vi "DealData.vi"(2 "mbfDealData":bool, 3 "ArrayIn":u8[](array[numeric]) format="0x%x") -> (0 "mu08BufSize":u8, 1 "Result":string[](array[string]))   [LabVIEW 2011]
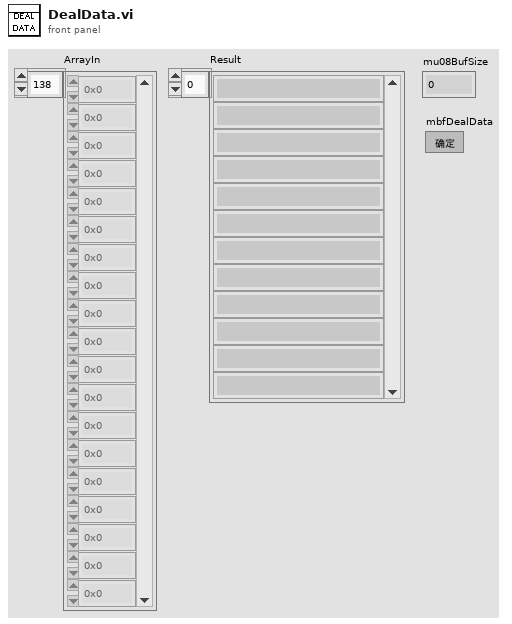
[diagram p1: front panel]
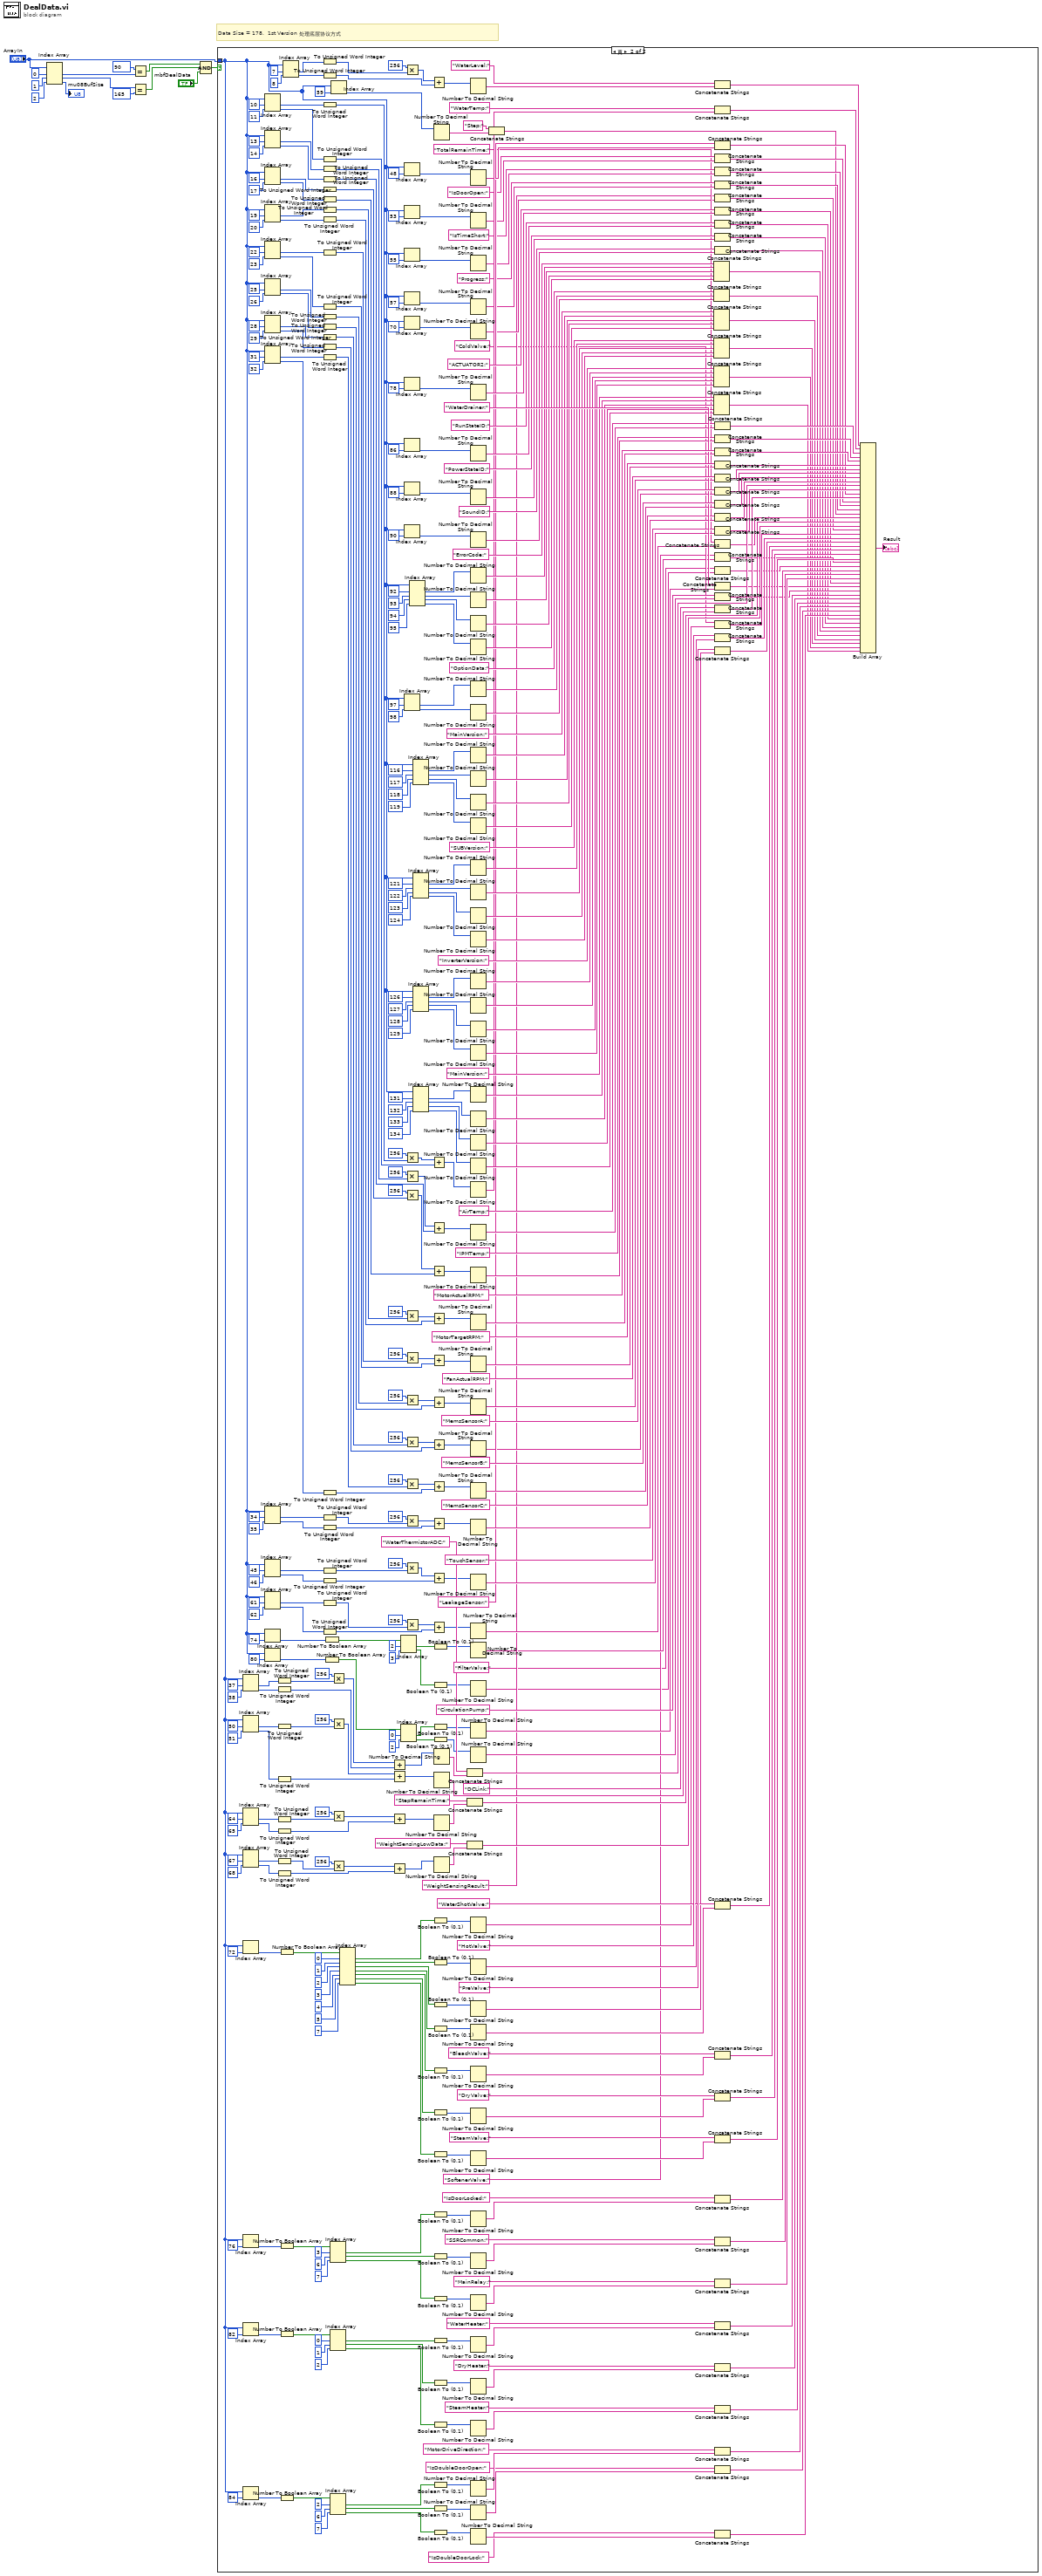
[diagram p0: block diagram]
diagram:
  # "Data Size = 178,  1st Version 处理底层协议方式"
  n1 = Index Array(array="ArrayIn", index #1=0 ("索引"), index #2=1 ("索引"), index #3=2 ("索引")) -> (element #1=w11:u8, element #2=w8:u8, element #3=→"mu08BufSize":u8)
  n2 = Equal?(x=u8 90, y=w11) -> (x = y?=w7:bool)
  n3 = Equal?(x=w8, y=u8 165) -> (x = y?=w6:bool)
  n4 = Compound Arithmetic op=AND(w7, w6, "mbfDealData") -> (w4:bool)
  n5 = case shown="真" w4 {
    tunnel: "ArrayIn" -> [_ w65]
    frame False {
    }
    frame True {
      n6 = Index Array(array=w65, index #1=37 ("索引"), index #2=38 ("索引")) -> (element #1=w361:u8, element #2=w360:u8)
      n7 = Index Array(array=w65, index #1=50 ("索引"), index #2=51 ("索引")) -> (element #1=w339:u8, element #2=w338:u8)
      n8 = Index Array(array=w65, index #1=64 ("索引"), index #2=65 ("索引")) -> (element #1=w305:u8, element #2=w304:u8)
      n9 = Index Array(array=w65, index #1=67 ("索引"), index #2=68 ("索引")) -> (element #1=w294:u8, element #2=w293:u8)
      n10 = Index Array(array=w65, index=72 ("索引")) -> (element=w287:u8)
      n11 = Index Array(array=w65, index=76 ("索引")) -> (element=w259:u8)
      n12 = Index Array(array=w65, index=82 ("索引")) -> (element=w224:u8)
      n13 = Index Array(array=w65, index=84 ("索引")) -> (element=w173:u8)
      n14 = Index Array(array=w65, index #1=10 ("索引"), index #2=11 ("索引")) -> (element #1=w460:u8, element #2=w457:u8)
      n15 = Index Array(array=w65, index #1=13 ("索引"), index #2=14 ("索引")) -> (element #1=w445:u8, element #2=w444:u8)
      n16 = Index Array(array=w65, index #1=16 ("索引"), index #2=17 ("索引")) -> (element #1=w426:u8, element #2=w425:u8)
      n17 = Index Array(array=w65, index #1=19 ("索引"), index #2=20 ("索引")) -> (element #1=w427:u8, element #2=w424:u8)
      n18 = Index Array(array=w65, index #1=22 ("索引"), index #2=23 ("索引")) -> (element #1=w414:u8, element #2=w413:u8)
      n19 = Index Array(array=w65, index #1=25 ("索引"), index #2=26 ("索引")) -> (element #1=w403:u8, element #2=w402:u8)
      n20 = Index Array(array=w65, index #1=28 ("索引"), index #2=29 ("索引")) -> (element #1=w392:u8, element #2=w391:u8)
      n21 = Index Array(array=w65, index #1=31 ("索引"), index #2=32 ("索引")) -> (element #1=w372:u8, element #2=w373:u8)
      n22 = Index Array(array=w65, index #1=34 ("索引"), index #2=35 ("索引")) -> (element #1=w369:u8, element #2=w370:u8)
      n23 = Index Array(array=w65, index #1=45 ("索引"), index #2=46 ("索引")) -> (element #1=w349:u8, element #2=w348:u8)
      n24 = Index Array(array=w65, index #1=61 ("索引"), index #2=62 ("索引")) -> (element #1=w316:u8, element #2=w315:u8)
      n25 = Index Array(array=w65, index=74 ("索引")) -> (element=w201:u8)
      n26 = Index Array(array=w65, index=80 ("索引")) -> (element=w237:u8)
      n27 = To Unsigned Word Integer(number=w361) -> (unsigned 16bit integer=w365:u16)
      n28 = To Unsigned Word Integer(number=w360) -> (unsigned 16bit integer=w363:u16)
      n29 = To Unsigned Word Integer(number=w339) -> (unsigned 16bit integer=w342:u16)
      n30 = To Unsigned Word Integer(number=w338) -> (unsigned 16bit integer=w341:u16)
      n31 = To Unsigned Word Integer(number=w305) -> (unsigned 16bit integer=w311:u16)
      n32 = To Unsigned Word Integer(number=w304) -> (unsigned 16bit integer=w310:u16)
      n33 = To Unsigned Word Integer(number=w294) -> (unsigned 16bit integer=w300:u16)
      n34 = To Unsigned Word Integer(number=w293) -> (unsigned 16bit integer=w299:u16)
      n35 = Number To Boolean Array(number=w287) -> (Boolean array=w286:bool[])
      n36 = Number To Boolean Array(number=w259) -> (Boolean array=w256:bool[])
      n37 = Number To Boolean Array(number=w224) -> (Boolean array=w223:bool[])
      n38 = Number To Boolean Array(number=w173) -> (Boolean array=w177:bool[])
      n39 = Index Array(array=w65, index #1=7 ("索引"), index #2=8 ("索引")) -> (element #1=w463:u8, element #2=w461:u8)
      n40 = To Unsigned Word Integer(number=w463) -> (unsigned 16bit integer=w464:u16)
      n41 = To Unsigned Word Integer(number=w461) -> (unsigned 16bit integer=w462:u16)
      n42 = To Unsigned Word Integer(number=w460) -> (unsigned 16bit integer=w459:u16)
      n43 = To Unsigned Word Integer(number=w457) -> (unsigned 16bit integer=w456:u16)
      n44 = To Unsigned Word Integer(number=w445) -> (unsigned 16bit integer=w450:u16)
      n45 = To Unsigned Word Integer(number=w444) -> (unsigned 16bit integer=w448:u16)
      n46 = To Unsigned Word Integer(number=w426) -> (unsigned 16bit integer=w440:u16)
      n47 = To Unsigned Word Integer(number=w425) -> (unsigned 16bit integer=w438:u16)
      n48 = To Unsigned Word Integer(number=w427) -> (unsigned 16bit integer=w432:u16)
      n49 = To Unsigned Word Integer(number=w424) -> (unsigned 16bit integer=w430:u16)
      n50 = To Unsigned Word Integer(number=w414) -> (unsigned 16bit integer=w419:u16)
      n51 = To Unsigned Word Integer(number=w413) -> (unsigned 16bit integer=w417:u16)
      n52 = To Unsigned Word Integer(number=w403) -> (unsigned 16bit integer=w408:u16)
      n53 = To Unsigned Word Integer(number=w402) -> (unsigned 16bit integer=w406:u16)
      n54 = To Unsigned Word Integer(number=w392) -> (unsigned 16bit integer=w397:u16)
      n55 = To Unsigned Word Integer(number=w391) -> (unsigned 16bit integer=w395:u16)
      n56 = To Unsigned Word Integer(number=w372) -> (unsigned 16bit integer=w386:u16)
      n57 = To Unsigned Word Integer(number=w373) -> (unsigned 16bit integer=w384:u16)
      n58 = To Unsigned Word Integer(number=w369) -> (unsigned 16bit integer=w377:u16)
      n59 = To Unsigned Word Integer(number=w370) -> (unsigned 16bit integer=w375:u16)
      n60 = To Unsigned Word Integer(number=w349) -> (unsigned 16bit integer=w354:u16)
      n61 = To Unsigned Word Integer(number=w348) -> (unsigned 16bit integer=w352:u16)
      n62 = To Unsigned Word Integer(number=w316) -> (unsigned 16bit integer=w322:u16)
      n63 = To Unsigned Word Integer(number=w315) -> (unsigned 16bit integer=w321:u16)
      n64 = Number To Boolean Array(number=w201) -> (Boolean array=w200:bool[])
      n65 = Number To Boolean Array(number=w237) -> (Boolean array=w236:bool[])
      n66 = Index Array(array=w256, index #1=3 ("索引"), index #2=6 ("索引"), index #3=7 ("索引")) -> (element #1=w254:bool, element #2=w253:bool, element #3=w252:bool)
      n67 = Index Array(array=w223, index #1=0 ("索引"), index #2=1 ("索引"), index #3=2 ("索引")) -> (element #1=w218:bool, element #2=w217:bool, element #3=w184:bool)
      n68 = Index Array(array=w177, index #1=2 ("索引"), index #2=6 ("索引"), index #3=7 ("索引")) -> (element #1=w169:bool, element #2=w168:bool, element #3=w167:bool)
      n69 = Index Array(array=w65, index=59 ("索引")) -> (element=w63:u8)
      n70 = Multiply(x=u16 256, y=w365) -> (x*y=w364:u16)
      n71 = Multiply(x=u16 256, y=w342) -> (x*y=w337:u16)
      n72 = Multiply(x=u16 256, y=w311) -> (x*y=w308:u16)
      n73 = Multiply(x=u16 256, y=w300) -> (x*y=w297:u16)
      n74 = Index Array(array=w286, index #1=0 ("索引"), index #2=1 ("索引"), index #3=2 ("索引"), index #4=3 ("索引"), index #5=4 ("索引"), index #6=5 ("索引"), index #7=7 ("索引")) -> (element #1=w276:bool, element #2=w275:bool, element #3=w274:bool, element #4=w273:bool, element #5=w272:bool, element #6=w209:bool, element #7=w208:bool)
      n75 = Add(x=w364, y=w363) -> (x+y=w362:u16)
      n76 = Add(x=w337, y=w341) -> (x+y=w336:u16)
      n77 = Add(x=w308, y=w310) -> (x+y=w307:u16)
      n78 = Add(x=w297, y=w299) -> (x+y=w296:u16)
      n79 = Index Array(array=w200, index #1=2 ("索引"), index #2=3 ("索引")) -> (element #1=w197:bool, element #2=w196:bool)
      n80 = Index Array(array=w236, index #1=0 ("索引"), index #2=2 ("索引")) -> (element #1=w233:bool, element #2=w232:bool)
      n81 = Index Array(array=w65, index=48 ("索引")) -> (element=w62:u8)
      n82 = Index Array(array=w65, index=53 ("索引")) -> (element=w334:u8)
      n83 = Index Array(array=w65, index=55 ("索引")) -> (element=w331:u8)
      n84 = Index Array(array=w65, index=57 ("索引")) -> (element=w328:u8)
      n85 = Index Array(array=w65, index=70 ("索引")) -> (element=w290:u8)
      n86 = Index Array(array=w65, index=78 ("索引")) -> (element=w239:u8)
      n87 = Index Array(array=w65, index=86 ("索引")) -> (element=w156:u8)
      n88 = Index Array(array=w65, index=88 ("索引")) -> (element=w151:u8)
      n89 = Index Array(array=w65, index=90 ("索引")) -> (element=w144:u8)
      n90 = Index Array(array=w65, index #1=97 ("索引"), index #2=98 ("索引")) -> (element #1=w123:u8, element #2=w122:u8)
      n91 = Multiply(x=u16 256, y=w464) -> (x*y=w470:u16)
      n92 = Multiply(x=u16 256, y=w459) -> (x*y=w458:u16)
      n93 = Multiply(x=u16 256, y=w450) -> (x*y=w449:u16)
      n94 = Multiply(x=u16 256, y=w440) -> (x*y=w439:u16)
      n95 = Multiply(x=u16 256, y=w432) -> (x*y=w431:u16)
      n96 = Multiply(x=u16 256, y=w419) -> (x*y=w418:u16)
      n97 = Multiply(x=u16 256, y=w408) -> (x*y=w407:u16)
      n98 = Multiply(x=u16 256, y=w397) -> (x*y=w396:u16)
      n99 = Multiply(x=u16 256, y=w386) -> (x*y=w385:u16)
      n100 = Multiply(x=u16 256, y=w377) -> (x*y=w376:u16)
      n101 = Multiply(x=u16 256, y=w354) -> (x*y=w353:u16)
      n102 = Multiply(x=u16 256, y=w322) -> (x*y=w319:u16)
      n103 = Index Array(array=w65, index #1=92 ("索引"), index #2=93 ("索引"), index #3=94 ("索引"), index #4=95 ("索引")) -> (element #1=w138:u8, element #2=w137:u8, element #3=w136:u8, element #4=w135:u8)
      n104 = Index Array(array=w65, index #1=116 ("索引"), index #2=117 ("索引"), index #3=118 ("索引"), index #4=119 ("索引")) -> (element #1=w115:u8, element #2=w114:u8, element #3=w111:u8, element #4=w110:u8)
      n105 = Index Array(array=w65, index #1=121 ("索引"), index #2=122 ("索引"), index #3=123 ("索引"), index #4=124 ("索引")) -> (element #1=w97:u8, element #2=w96:u8, element #3=w95:u8, element #4=w94:u8)
      n106 = Index Array(array=w65, index #1=126 ("索引"), index #2=127 ("索引"), index #3=128 ("索引"), index #4=129 ("索引")) -> (element #1=w87:u8, element #2=w86:u8, element #3=w83:u8, element #4=w82:u8)
      n107 = Index Array(array=w65, index #1=131 ("索引"), index #2=132 ("索引"), index #3=133 ("索引"), index #4=134 ("索引")) -> (element #1=w73:u8, element #2=w72:u8, element #3=w69:u8, element #4=w68:u8)
      n108 = Add(x=w470, y=w462) -> (x+y=w61:u16)
      n109 = Add(x=w458, y=w456) -> (x+y=w455:u16)
      n110 = Add(x=w449, y=w448) -> (x+y=w447:u16)
      n111 = Add(x=w439, y=w438) -> (x+y=w437:u16)
      n112 = Add(x=w431, y=w430) -> (x+y=w429:u16)
      n113 = Add(x=w418, y=w417) -> (x+y=w416:u16)
      n114 = Add(x=w407, y=w406) -> (x+y=w405:u16)
      n115 = Add(x=w396, y=w395) -> (x+y=w394:u16)
      n116 = Add(x=w385, y=w384) -> (x+y=w383:u16)
      n117 = Add(x=w376, y=w375) -> (x+y=w374:u16)
      n118 = Add(x=w353, y=w352) -> (x+y=w351:u16)
      n119 = Add(x=w319, y=w321) -> (x+y=w318:u16)
      n120 = Boolean To (0,1)(Boolean=w197) -> (0, 1=w195:i16)
      n121 = Boolean To (0,1)(Boolean=w196) -> (0, 1=w194:i16)
      n122 = Boolean To (0,1)(Boolean=w233) -> (0, 1=w231:i16)
      n123 = Boolean To (0,1)(Boolean=w232) -> (0, 1=w230:i16)
      n124 = Boolean To (0,1)(Boolean=w276) -> (0, 1=w271:i16)
      n125 = Boolean To (0,1)(Boolean=w275) -> (0, 1=w270:i16)
      n126 = Boolean To (0,1)(Boolean=w274) -> (0, 1=w269:i16)
      n127 = Boolean To (0,1)(Boolean=w273) -> (0, 1=w268:i16)
      n128 = Boolean To (0,1)(Boolean=w272) -> (0, 1=w267:i16)
      n129 = Boolean To (0,1)(Boolean=w209) -> (0, 1=w207:i16)
      n130 = Boolean To (0,1)(Boolean=w208) -> (0, 1=w206:i16)
      n131 = Boolean To (0,1)(Boolean=w254) -> (0, 1=w251:i16)
      n132 = Boolean To (0,1)(Boolean=w253) -> (0, 1=w250:i16)
      n133 = Boolean To (0,1)(Boolean=w252) -> (0, 1=w249:i16)
      n134 = Boolean To (0,1)(Boolean=w218) -> (0, 1=w220:i16)
      n135 = Boolean To (0,1)(Boolean=w217) -> (0, 1=w219:i16)
      n136 = Boolean To (0,1)(Boolean=w184) -> (0, 1=w183:i16)
      n137 = Boolean To (0,1)(Boolean=w169) -> (0, 1=w172:i16)
      n138 = Boolean To (0,1)(Boolean=w168) -> (0, 1=w171:i16)
      n139 = Boolean To (0,1)(Boolean=w167) -> (0, 1=w170:i16)
      n140 = Number To Decimal String(number=w63) -> (decimal integer string=w33:string)  [unwired: 1 in]
      n141 = Number To Decimal String(number=w362) -> (decimal integer string=w46:string)  [unwired: 1 in]
      n142 = Number To Decimal String(number=w336) -> (decimal integer string=w42:string)  [unwired: 1 in]
      n143 = Number To Decimal String(number=w307) -> (decimal integer string=w30:string)  [unwired: 1 in]
      n144 = Number To Decimal String(number=w296) -> (decimal integer string=w29:string)  [unwired: 1 in]
      n145 = Concatenate Strings("WaterThermistorADC:", w46) -> (w358:string)
      n146 = Concatenate Strings("StepRemainTime:", w30) -> (w303:string)
      n147 = Concatenate Strings("WeightSensingLowData:", w29) -> (w292:string)
      n148 = Number To Decimal String(number=w61) -> (decimal integer string=w60:string)  [unwired: 1 in]
      n149 = Number To Decimal String(number=w62) -> (decimal integer string=w44:string)  [unwired: 1 in]
      n150 = Number To Decimal String(number=w334) -> (decimal integer string=w40:string)  [unwired: 1 in]
      n151 = Number To Decimal String(number=w331) -> (decimal integer string=w38:string)  [unwired: 1 in]
      n152 = Number To Decimal String(number=w328) -> (decimal integer string=w36:string)  [unwired: 1 in]
      n153 = Number To Decimal String(number=w290) -> (decimal integer string=w28:string)  [unwired: 1 in]
      n154 = Number To Decimal String(number=w239) -> (decimal integer string=w240:string)  [unwired: 1 in]
      n155 = Number To Decimal String(number=w156) -> (decimal integer string=w154:string)  [unwired: 1 in]
      n156 = Number To Decimal String(number=w151) -> (decimal integer string=w150:string)  [unwired: 1 in]
      n157 = Number To Decimal String(number=w144) -> (decimal integer string=w146:string)  [unwired: 1 in]
      n158 = Number To Decimal String(number=w138) -> (decimal integer string=w133:string)  [unwired: 1 in]
      n159 = Number To Decimal String(number=w137) -> (decimal integer string=w132:string)  [unwired: 1 in]
      n160 = Number To Decimal String(number=w136) -> (decimal integer string=w131:string)  [unwired: 1 in]
      n161 = Number To Decimal String(number=w135) -> (decimal integer string=w130:string)  [unwired: 1 in]
      n162 = Number To Decimal String(number=w123) -> (decimal integer string=w125:string)  [unwired: 1 in]
      n163 = Number To Decimal String(number=w122) -> (decimal integer string=w124:string)  [unwired: 1 in]
      n164 = Number To Decimal String(number=w115) -> (decimal integer string=w117:string)  [unwired: 1 in]
      n165 = Number To Decimal String(number=w114) -> (decimal integer string=w116:string)  [unwired: 1 in]
      n166 = Number To Decimal String(number=w111) -> (decimal integer string=w109:string)  [unwired: 1 in]
      n167 = Number To Decimal String(number=w110) -> (decimal integer string=w108:string)  [unwired: 1 in]
      n168 = Number To Decimal String(number=w97) -> (decimal integer string=w103:string)  [unwired: 1 in]
      n169 = Number To Decimal String(number=w96) -> (decimal integer string=w102:string)  [unwired: 1 in]
      n170 = Number To Decimal String(number=w95) -> (decimal integer string=w99:string)  [unwired: 1 in]
      n171 = Number To Decimal String(number=w94) -> (decimal integer string=w98:string)  [unwired: 1 in]
      n172 = Number To Decimal String(number=w87) -> (decimal integer string=w89:string)  [unwired: 1 in]
      n173 = Number To Decimal String(number=w86) -> (decimal integer string=w88:string)  [unwired: 1 in]
      n174 = Number To Decimal String(number=w83) -> (decimal integer string=w81:string)  [unwired: 1 in]
      n175 = Number To Decimal String(number=w82) -> (decimal integer string=w80:string)  [unwired: 1 in]
      n176 = Number To Decimal String(number=w73) -> (decimal integer string=w75:string)  [unwired: 1 in]
      n177 = Number To Decimal String(number=w72) -> (decimal integer string=w74:string)  [unwired: 1 in]
      n178 = Number To Decimal String(number=w69) -> (decimal integer string=w67:string)  [unwired: 1 in]
      n179 = Number To Decimal String(number=w68) -> (decimal integer string=w66:string)  [unwired: 1 in]
      n180 = Number To Decimal String(number=w455) -> (decimal integer string=w59:string)  [unwired: 1 in]
      n181 = Number To Decimal String(number=w447) -> (decimal integer string=w57:string)  [unwired: 1 in]
      n182 = Number To Decimal String(number=w437) -> (decimal integer string=w55:string)  [unwired: 1 in]
      n183 = Number To Decimal String(number=w429) -> (decimal integer string=w54:string)  [unwired: 1 in]
      n184 = Number To Decimal String(number=w416) -> (decimal integer string=w52:string)  [unwired: 1 in]
      n185 = Number To Decimal String(number=w405) -> (decimal integer string=w51:string)  [unwired: 1 in]
      n186 = Number To Decimal String(number=w394) -> (decimal integer string=w34:string)  [unwired: 1 in]
      n187 = Number To Decimal String(number=w383) -> (decimal integer string=w50:string)  [unwired: 1 in]
      n188 = Number To Decimal String(number=w374) -> (decimal integer string=w47:string)  [unwired: 1 in]
      n189 = Number To Decimal String(number=w351) -> (decimal integer string=w45:string)  [unwired: 1 in]
      n190 = Number To Decimal String(number=w318) -> (decimal integer string=w32:string)  [unwired: 1 in]
      n191 = Number To Decimal String(number=w195) -> (decimal integer string=w18:string)  [unwired: 1 in]
      n192 = Number To Decimal String(number=w194) -> (decimal integer string=w16:string)  [unwired: 1 in]
      n193 = Number To Decimal String(number=w231) -> (decimal integer string=w227:string)  [unwired: 1 in]
      n194 = Number To Decimal String(number=w230) -> (decimal integer string=w226:string)  [unwired: 1 in]
      n195 = Number To Decimal String(number=w271) -> (decimal integer string=w26:string)  [unwired: 1 in]
      n196 = Number To Decimal String(number=w270) -> (decimal integer string=w24:string)  [unwired: 1 in]
      n197 = Number To Decimal String(number=w269) -> (decimal integer string=w23:string)  [unwired: 1 in]
      n198 = Number To Decimal String(number=w268) -> (decimal integer string=w22:string)  [unwired: 1 in]
      n199 = Number To Decimal String(number=w267) -> (decimal integer string=w21:string)  [unwired: 1 in]
      n200 = Number To Decimal String(number=w207) -> (decimal integer string=w20:string)  [unwired: 1 in]
      n201 = Number To Decimal String(number=w206) -> (decimal integer string=w19:string)  [unwired: 1 in]
      n202 = Number To Decimal String(number=w251) -> (decimal integer string=w245:string)  [unwired: 1 in]
      n203 = Number To Decimal String(number=w250) -> (decimal integer string=w244:string)  [unwired: 1 in]
      n204 = Number To Decimal String(number=w249) -> (decimal integer string=w243:string)  [unwired: 1 in]
      n205 = Number To Decimal String(number=w220) -> (decimal integer string=w214:string)  [unwired: 1 in]
      n206 = Number To Decimal String(number=w219) -> (decimal integer string=w213:string)  [unwired: 1 in]
      n207 = Number To Decimal String(number=w183) -> (decimal integer string=w181:string)  [unwired: 1 in]
      n208 = Number To Decimal String(number=w172) -> (decimal integer string=w165:string)  [unwired: 1 in]
      n209 = Number To Decimal String(number=w171) -> (decimal integer string=w164:string)  [unwired: 1 in]
      n210 = Number To Decimal String(number=w170) -> (decimal integer string=w162:string)  [unwired: 1 in]
      n211 = Concatenate Strings("Step:", w33) -> (w324:string)
      n212 = Concatenate Strings("ErrorCode:", w133, w132, w131, w130) -> (w129:string)
      n213 = Concatenate Strings("OptionData:", w125, w124) -> (w121:string)
      n214 = Concatenate Strings("MainVersion:", w117, w116, w109, w108) -> (w107:string)
      n215 = Concatenate Strings("SUBVersion:", w103, w102, w99, w98) -> (w93:string)
      n216 = Concatenate Strings("InverterVersion:", w89, w88, w81, w80) -> (w79:string)
      n217 = Concatenate Strings("MainVersion:", w75, w74, w67, w66) -> (w64:string)
      n218 = Concatenate Strings("WaterLevel:", w60) -> (w468:string)
      n219 = Concatenate Strings("WaterTemp:", w59) -> (w454:string)
      n220 = Concatenate Strings("LeakageSensor:", w44) -> (w346:string)
      n221 = Concatenate Strings("IsDoorOpen:", w40) -> (w333:string)
      n222 = Concatenate Strings("IsTimeShort:", w38) -> (w330:string)
      n223 = Concatenate Strings("Progress:", w36) -> (w327:string)
      n224 = Concatenate Strings("WeightSensingResult:", w28) -> (w289:string)
      n225 = Concatenate Strings("ACTUATOR2:", w240) -> (w188:string)
      n226 = Concatenate Strings("RunStateID:", w154) -> (w153:string)
      n227 = Concatenate Strings("PowerStateID:", w150) -> (w148:string)
      n228 = Concatenate Strings("SoundID:", w146) -> (w143:string)
      n229 = Concatenate Strings("AirTemp:", w57) -> (w446:string)
      n230 = Concatenate Strings("IPMTemp:", w55) -> (w436:string)
      n231 = Concatenate Strings("MotorActualRPM:", w54) -> (w423:string)
      n232 = Concatenate Strings("MotorTargetRPM:", w52) -> (w412:string)
      n233 = Concatenate Strings("FanActualRPM:", w51) -> (w401:string)
      n234 = Concatenate Strings("MemsSensorA:", w34) -> (w390:string)
      n235 = Concatenate Strings("MemsSensorB:", w50) -> (w381:string)
      n236 = Concatenate Strings("MemsSensorC:", w47) -> (w371:string)
      n237 = Concatenate Strings("TouchSensor:", w45) -> (w350:string)
      n238 = Concatenate Strings("TotalRemainTime:", w32) -> (w314:string)
      n239 = Concatenate Strings("SoftenerValve:", w18) -> (w193:string)
      n240 = Concatenate Strings("FilterValve:", w16) -> (w192:string)
      n241 = Concatenate Strings("WaterDrainer:", w227) -> (w187:string)
      n242 = Concatenate Strings("CirculationPump:", w226) -> (w186:string)
      n243 = Concatenate Strings("DCLink:", w42) -> (w344:string)
      n244 = Concatenate Strings("ColdValve:", w26) -> (w266:string)
      n245 = Concatenate Strings("HotValve:", w24) -> (w265:string)
      n246 = Concatenate Strings("PreValve:", w23) -> (w264:string)
      n247 = Concatenate Strings("WaterShotValve:", w22) -> (w263:string)
      n248 = Concatenate Strings("BleachValve:", w21) -> (w262:string)
      n249 = Concatenate Strings("DryValve:", w20) -> (w203:string)
      n250 = Concatenate Strings("SteamValve:", w19) -> (w202:string)
      n251 = Concatenate Strings("IsDoorLocked:", w245) -> (w191:string)
      n252 = Concatenate Strings("SSRCommon:", w244) -> (w190:string)
      n253 = Concatenate Strings("MainRelay:", w243) -> (w189:string)
      n254 = Concatenate Strings("WaterHeater:", w214) -> (w180:string)
      n255 = Concatenate Strings("DryHeater:", w213) -> (w179:string)
      n256 = Concatenate Strings("SteamHeater:", w181) -> (w178:string)
      n257 = Concatenate Strings("MotorDriveDirection:", w165) -> (w160:string)
      n258 = Concatenate Strings("IsDoubleDoorOpen:", w164) -> (w159:string)
      n259 = Concatenate Strings("IsDoubleDoorLock:", w162) -> (w158:string)
      n260 = Build Array(w468, w454, w446, w436, w423, w412, w401, w390, w381, w371, w358, w350, w346, w344, w333, w330, w327, w324, w314, w303, w292, w289, w266, w265, w264, w263, w262, w203, w202, w193, w192, w191, w190, w189, w188, w187, w186, w180, w179, w178, w160, w159, w158, w153, w148, w143, w129, w121, w107, w93, w79, w64) -> (→"Result":string[])
    }
  }
